vi "FTW-SQLite-Backup-Async.vi"(0 "SQLite Connector":refnum<class "FTW-SQLite-Connector.lvclass">, 5 "Destination Database Filepath":path, 11 "error in":errorcluster) -> (4 "SQLite Connector out":refnum<class "FTW-SQLite-Connector.lvclass">, 15 "error out":errorcluster)   [LabVIEW 2013, in "FTW-SQLite-Connector.lvclass"]
uses:
  FTW-SQLite-Connector.lvclass
  FTW-SQLite-AccessMode.ctl
  FTW-SQLite-Backup-Worker.vi
  FTW-SQLite-AsyncOperation.ctl
panel:
  out "Backup Progress":refnum<event-registration>
  # "Inputs"
  # "Outputs"
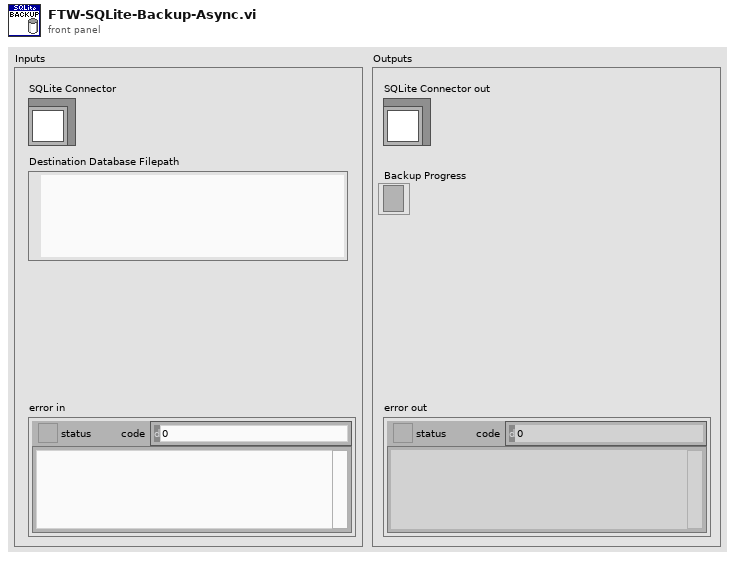
[diagram p1: front panel]
types:
  T1 = typedef "FTW-SQLite-Connector.lvclass/FTW-SQLite-AccessMode.ctl" = enum16{"Read", "Read/Write", "Read/Write/Create"}
  T2 = typedef "FTW-SQLite-Connector.lvclass/FTW-SQLite-AsyncOperation.ctl" = cluster{"Connector":refnum<class "FTW-SQLite-Connector.lvclass">, "Progress (0.0-100.0%)":dbl, "Time Elapsed (msec)":u32, "Estimated Time Remaining (msec)":u32}
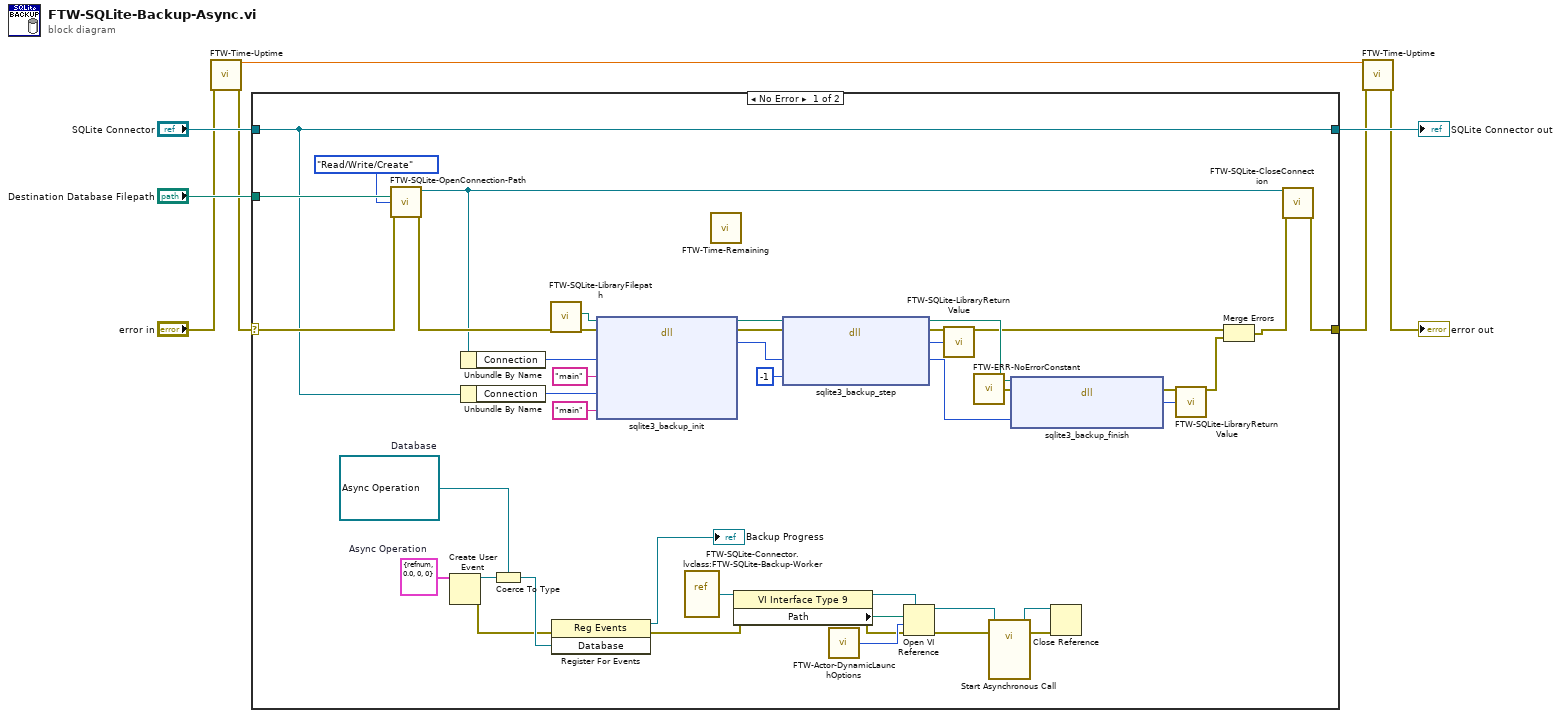
[diagram p0: block diagram]
diagram:
  n1 = call "FTW-Time-Uptime.vi"("error in"="error in") -> ("Current Uptime"=w4:dbl, "error out"=w5:errorcluster)  [unwired: 12 in, 1 out]
  n2 = case shown="No Error" w5 {
    selector: w5 -> [w52 w54]
    tunnel: "SQLite Connector" -> [w41 w55]
    tunnel: [w41 w55] -> w8
    tunnel: "Destination Database Filepath" -> [w53 _]
    tunnel: [w28 w54] -> w2
    frame No Error {
      w11 = T2 {"Connector"=refnum, "Progress (0.0-100.0%)"=0.0, "Time Elapsed (msec)"=0, "Estimated Time Remaining (msec)"=0}  # Async Operation
      w22 = refnum<user-event> refnum  # Database
      n3 = call "FTW-SQLite-OpenConnection-Path.vi"("Database Filepath"=w53, "Access Mode"=FTW-SQLite-AccessMode."Read/Write/Create", "error in"=w52) -> ("SQLite Connector"=w30:refnum<class "FTW-SQLite-Connector.lvclass">, "error out"=w51:errorcluster)  [unwired: 11 in]
      n4 = Create User Event(user event datatype=w11) -> (error in=w12:errorcluster, user event=w21:refnum<user-event>, error out=w20:errorcluster)
      n5 = Unbundle By Name(w30) -> ("Connection"=w43:u64)
      n6 = Unbundle By Name(w41) -> ("Connection"=w40:u64)
      n7 = Coerce To Type(0:w21, 1:w22) -> (2:w26:refnum<user-event>)
      n8 = call "FTW-SQLite-LibraryFilepath.vi"("error in"=w51) -> ("error out"=w44:errorcluster, "SQLite Library Filepath"=w45:path)  [unwired: 8 in, 1 out]
      n9 = register-events(error in=w20, w26) -> (reference out=→"Backup Progress":refnum<event-registration>, error out=w23:errorcluster)  [unwired: 1 in]
      n10 = dll-call lib="?" fn="sqlite3_backup_init"(path in=w45, error in=w44, "Destination Pointer"=w43, "Destination Name"="main", "Source Pointer"=w40, "Source Name"="main") -> (path out=w35:path, error out=w32:errorcluster, "Backup Object"=w34:u64)  [unwired: 5 in]
      n11 = vi-ref "FTW-SQLite-Connector.lvclass:FTW-SQLite-Backup-Worker.vi"() -> (w13:refnum<vi>)
      n12 = call "FTW-Time-Remaining.vi"() -> ()  [unwired: 11 in, 5 out]
      n13 = property class="VI Interface Type 9"(reference=w13, error in=w23) -> (reference out=w14:refnum<vi>, error out=w17:errorcluster, "Path"=w15:path)
      n14 = dll-call lib="?" fn="sqlite3_backup_step"(path in=w35, error in=w32, "Backup Object"=w34, "NumPages"=-1) -> (path out=w47:path, error out=w38:errorcluster, "Return Type"=w36:i32, "Backup Object"=w50:u64)  [unwired: 2 in]
      n15 = call "FTW-Actor-DynamicLaunchOptions.vi"() -> ("Open VI Ref Options"=w18:i32)  [unwired: 1 in]
      n16 = Open VI Reference(type specifier VI Refnum (for type only)=w14, vi path=w15, options=w18, error in (no error)=w17) -> (vi reference=w19:refnum<vi>, error out=w16:errorcluster)  [unwired: 2 in]
      n17 = call "FTW-SQLite-LibraryReturnValue.vi"("error in"=w38, "Return Value"=w36) -> ("error out"=w37:errorcluster)  [unwired: 13 in]
      n18 = call "FTW-ERR-NoErrorConstant.vi"() -> ("no error"=w33:errorcluster)
      n19 = call-by-ref "Start Asynchronous Call"(reference=w19, error in=w16) -> (reference out=w24:refnum<vi>, error out=w25:errorcluster)  [unwired: 4 in]
      n20 = dll-call lib="?" fn="sqlite3_backup_finish"(path in=w47, error in=w33, "Backup Object"=w50) -> (error out=w49:errorcluster, "Return Value"=w48:i32)  [unwired: 2 in, 1 out]
      n21 = Close Reference(reference=w24, error in (no error)=w25) -> ()  [unwired: 1 out]
      n22 = call "FTW-SQLite-LibraryReturnValue.vi"("error in"=w49, "Return Value"=w48) -> ("error out"=w46:errorcluster)  [unwired: 13 in]
      n23 = Merge Errors(w37, w46) -> (w29:errorcluster)
      n24 = call "FTW-SQLite-CloseConnection.vi"("SQLite Connector"=w30, "error in"=w29) -> ("error out"=w28:errorcluster)  [unwired: 13 in]
    }
    frame Error {
    }
  }
  "SQLite Connector out" <- w8
  n25 = call "FTW-Time-Uptime.vi"("Previous Uptime"=w4, "error in"=w2) -> ("Elapsed Time"=w1:dbl, "error out"=→"error out":errorcluster)  [unwired: 11 in, 1 out]
